vi "Configure Carrier Signal.vi"(0 "VISA resource name":refnum<visa-resource-name>, 1 "Frequency (10000000Hz)":dbl=10000000.0, 5 "Phase (0 Degrees)":dbl, 7 "LF Amplitude (0 dBm)":dbl, 9 "RF Amplitude (0 dBm)":dbl, 11 "error in (no error)":errorcluster) -> (4 "VISA resource name out":refnum<visa-resource-name>, 15 "error out":errorcluster)   [LabVIEW 2015, in "Stanford Research SG39x Series.lvlib"]
doc: "Configures the characteristics of the carrier signal."
uses:
  Stanford Research SG39x Series.lvlib
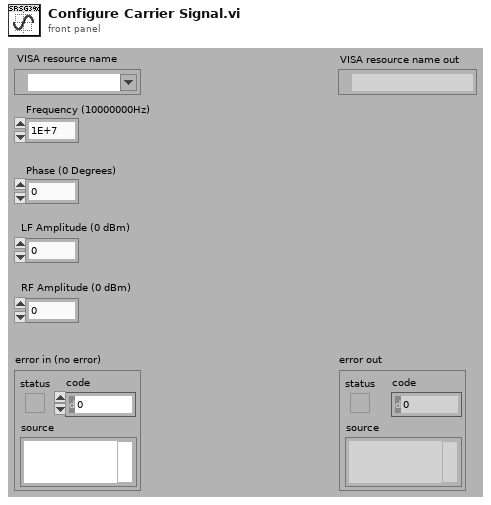
[diagram p1: front panel]
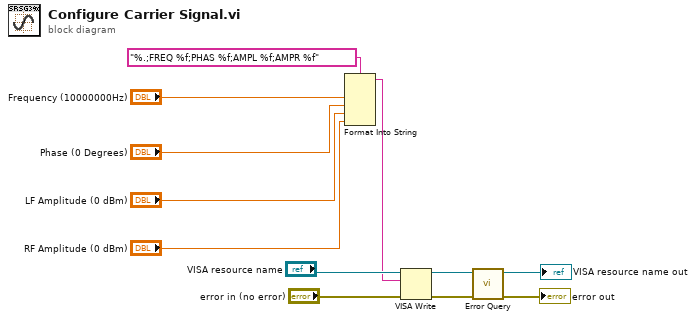
[diagram p0: block diagram]
diagram:
  n1 = Format Into String(format string="%.;FREQ %f;PHAS %f;AMPL %f;AMPR %f", "Frequency (10000000Hz)", "Phase (0 Degrees)", "LF Amplitude (0 dBm)", "RF Amplitude (0 dBm)") -> (resulting string=w5:string)  [unwired: 2 in, 1 out]
  n2 = VISA Write(VISA resource name="VISA resource name", write buffer=w5, error in (no error)="error in (no error)") -> (VISA resource name out=w4:refnum<visa-resource-name>, error out=w3:errorcluster)  [unwired: 1 out]
  n3 = call "Error Query.vi"("error in (no error)"=w3, "VISA resource name"=w4) -> ("error out"=→"error out":errorcluster, "VISA resource name out"=→"VISA resource name out":refnum<visa-resource-name>)  [unwired: 6 in, 2 out]
